vi "SPD.Set HV_Bias and Wait For Ready.vi"(7 "Continue":refnum<vi>, 8 "Error In":errorcluster, 10 "HV_Bias":dbl, 11 "SPD.Stand Ctrl in":T1 {"spdDeviceSession"."hidSPD.Controller"."HV_bias" format="%#_6p, V"; "spdDeviceSession"."hidSPD.Controller"."TSet" format="%#_6p, DegC"}) -> (0 "Error Out":errorcluster, 3 "SPD.Stand Ctrl out":T1 {"spdDeviceSession"."hidSPD.Controller"."HV_bias" format="%#_6p, V"; "spdDeviceSession"."hidSPD.Controller"."TSet" format="%#_6p, DegC"})   [LabVIEW 2018]
uses:
  typedefs/SPD.Stand Ctrl.ctl
  Instruments/SPD HID Interface/hidSPDLibForLabView/LibVIs/hidSPD Controls/hidSPD Device Session.ctl
  Instruments/SPD HID Interface/hidSPDLibForLabView/LibVIs/hidSPD Controls/hidSPD Controller.ctl
  Instruments/KC705 DevBoard/typedefs/DevB.Session.ctl
  Instruments/KeySight 53230A/typedefs/FreqC.Session.ctl
  Instruments/KeySight 8164B/KeySight 8164B LAN InstrLib/typedefs/KeySight 8164B control.ctl
  Instruments/LeCroy SDA830/typedefs/LeCroy.Session.ctl
  typedefs/SPD.Events.ctl
  <vilib>/Utility/config.llb/Config Data RefNum.ctl
  typedefs/SPD.Meas Result.ctl
  Instruments/SPD HID Interface/hidSPDLibForLabView/LibVIs/hidSPD Controls/hidSPD Controller Setup Report.ctl
  Instruments/SPD HID Interface/hidSPDLibForLabView/LibVIs/hidSPD Write Report/hidSPD Setup Controller.vi
  Instruments/SPD HID Interface/hidSPDLibForLabView/hidSPDLibForLabView.lvlib
  Instruments/KeySight 8164B/KeySight 8164B LAN InstrLib.lvlib
  <vilib>/Utility/config.llb/NI_LVConfig.lvlib
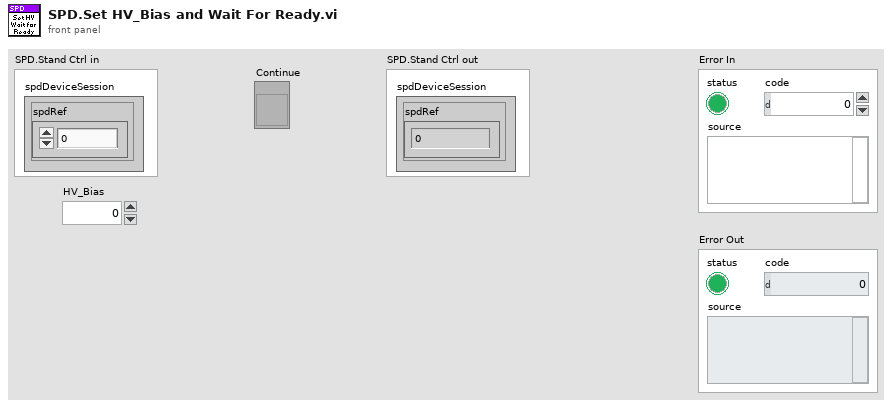
[diagram p1: front panel]
types:
  T1 = typedef "SPD.Stand Ctrl.ctl" = cluster{"spdDeviceSession":T2, "DevBSession":T4, "FreqCSession":T5, "8164BSession":T6, "LeCroySession":T7, "Events":T8, "configFile":T9, "SPD.Result":T10}
  T2 = typedef "hidSPDLibForLabView.lvlib/hidSPD Device Session.ctl" = cluster{"spdRef":u64, "connected":bool, "spdName":string, "hidSPD.Controller":T3}
  T3 = typedef "hidSPDLibForLabView.lvlib/hidSPD Controller.ctl" = cluster{"TSet":sgl, "HV_bias":sgl, "DDS_stb_code":u16}
  T4 = typedef "DevB.Session.ctl" = cluster{"DevBRef":refnum<visa-resource-name>, "connected":bool}
  T5 = typedef "FreqC.Session.ctl" = cluster{"FreqCRef":refnum<visa-resource-name>, "timeout":dbl, "connected":bool}
  T6 = typedef "KeySight 8164B LAN InstrLib.lvlib/KeySight 8164B control.ctl" = cluster{"Connection ID":refnum<k5>, "Connected":bool, "Info":string, "Slots Info":string[]}
  T7 = typedef "LeCroy.Session.ctl" = cluster{"LeCroySession":refnum<visa-resource-name>, "connected":bool}
  T8 = typedef "SPD.Events.ctl" = cluster{"DCRTest":refnum<user-event>, "Stop":refnum<user-event>}
  T9 = typedef "NI_LVConfig.lvlib/Config Data RefNum.ctl" = refnum<k1>
  T10 = typedef "SPD.Meas Result.ctl" = cluster{"HV_Bias":dbl[], "Stb_code":dbl[], "Temprature":dbl[], "Data":dbl[][][][]}
  T11 = typedef "hidSPDLibForLabView.lvlib/hidSPD Controller Setup Report.ctl" = cluster{"TSet":sgl, "HV_bias":sgl, "DDS_stb_code":u16, "SPD_reset":u16, "MCU_reset":u16}
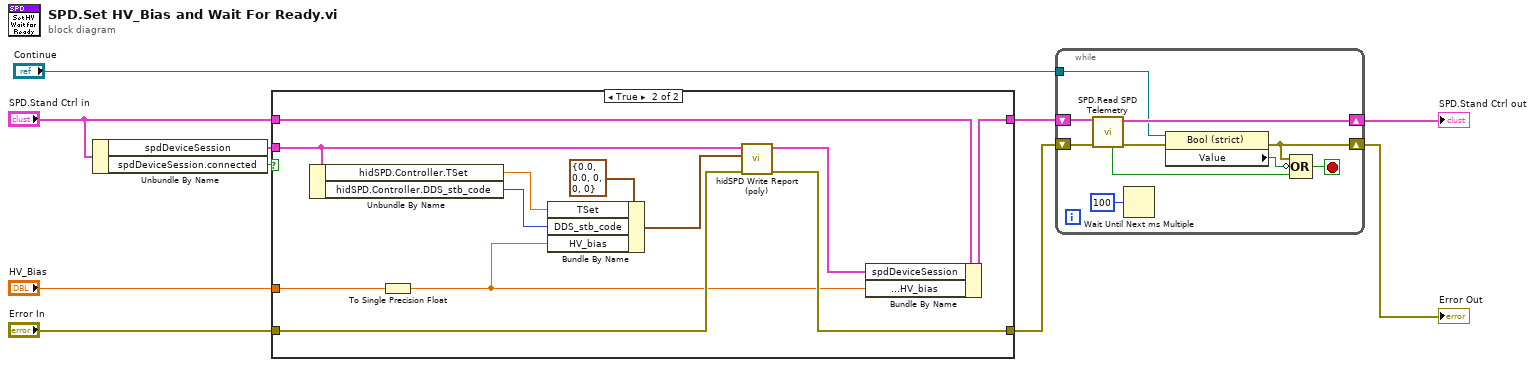
[diagram p0: block diagram]
diagram:
  n1 = Unbundle By Name("SPD.Stand Ctrl in") -> ("spdDeviceSession"=w10:T2, "spdDeviceSession.connected"=w9:bool)
  n2 = case shown="True" w9 {
    tunnel: w10 -> [_ w20]
    tunnel: "Error In" -> [w11 w22]
    tunnel: "SPD.Stand Ctrl in" -> [w12 w24]
    tunnel: [w12 w23] -> w5
    tunnel: [w11 w21] -> w4
    tunnel: "HV_Bias" -> [_ w16]
    frame False {
    }
    frame True {
      n3 = Unbundle By Name(w20) -> ("hidSPD.Controller.TSet"=w17:sgl, "hidSPD.Controller.DDS_stb_code"=w15:u16)
      n4 = To Single Precision Float(number=w16) -> (single precision float=w14:sgl)
      n5 = Bundle By Name(cluster=T11 {"TSet"=0.0, "HV_bias"=0.0, "DDS_stb_code"=0, "SPD_reset"=0, "MCU_reset"=0} ("hidSPD Controller Setup report"), "TSet"=w17, "DDS_stb_code"=w15, "HV_bias"=w14) -> (w18:T11)
      n6 = call-poly "hidSPD Write Report (poly).vi"("error in (no error)"=w22, "hidSPD Controller Setup report"=w18, "spdDevSession in"=w20) -> ("error out"=w21:errorcluster, "spdDevSession out"=w13:T2)  [unwired: 7 in]
      n7 = Bundle By Name(cluster=w24, "spdDeviceSession"=w13, "spdDeviceSession.hidSPD.Controller.HV_bias"=w14) -> (w23:T1)
    }
  }
  n8 = while {
    shift-right: [w27] -> w2
    shift-left: w4 -> [w33]
    shift-right: [w31] -> w3
    shift-left: w5 -> [w34]
    tunnel: "Continue" -> [w30]
    stop <- w29 stop-if-true
    n9 = call "SPD.Read SPD Telemetry.vi"("Error In"=w33, "SPD.Stand Ctrl in"=w34) -> ("Error Out"=w28:errorcluster, "SPD.Stand Ctrl out"=w31:T1, "Ready"=w25:bool)  [unwired: 5 in, 2 out]
    n10 = Wait Until Next ms Multiple(millisecond multiple=u32 100) -> ()  [unwired: 1 out]
    n11 = property class="Bool (strict)"(reference=w30, error in=w28) -> (error out=w27:errorcluster, "Value"=w26:bool)  [unwired: 1 out]
    n12 = Compound Arithmetic op=OR(w27, invert w26, w25) -> (w29:bool)
  }
  "SPD.Stand Ctrl out" <- w3
  "Error Out" <- w2
